vi "AH Bridge Update Int Cal.vi"(8 "error in (no error)":errorcluster, 11 "VISA resource name":refnum<visa-resource-name>) -> (0 "error out":errorcluster, 1 "Cal Done time string":string, 2 "Start time string":string, 3 "dup VISA Session":refnum<visa-resource-name>)   [LabVIEW 2025]
doc: "routine to calibrate the AH 2700 Bridge using the internal standard\nWaits for command ready status and stores calibration data, updating the calibration due date.\n\nScott Hannahs, NHMFL December 2023\n<sth@magnet.fsu.edu>\nAuthor: Scott Hannahs <sth@magnet.fsu.edu>\n\nThis software is licensed for use under the “MIT License\"\nCopyright (c) 2025 Scott Hannahs, sth@sth@magnet.sthnet.net\n\nPermission is hereby granted, free of charge, to any person obtaining a copy of this software and associated documentation files (the \"Software\"), to deal in the Software without restriction, including without limitation the rights to use, copy, modify, merge, publish, distribute, sublicense, and/or sell copies of the Software, and to permit persons to whom the Software is furnished to do so, subject to the following conditions: The above copyright notice and this permission notice shall be included in all copies or substantial portions of the Software.\n\nTHE SOFTWARE IS PROVIDED \"AS IS\", WITHOUT WARRANTY OF ANY KIND, EXPRESS OR IMPLIED, INCLUDING BUT NOT LIMITED TO THE WARRANTIES OF MERCHANTABILITY, FITNESS FOR A PARTICULAR PURPOSE AND NONINFRINGEMENT. IN NO EVENT SHALL THE AUTHORS OR COPYRIGHT HOLDERS BE LIABLE FOR ANY CLAIM, DAMAGES OR OTHER LIABILITY, WHETHER IN AN ACTION OF CONTRACT, TORT OR OTHERWISE, ARISING FROM, OUT OF OR IN CONNECTION WITH THE SOFTWARE OR THE USE OR OTHER DEALINGS IN THE SOFTWARE."
panel:
  out "status byte":u16 format="%.0b"
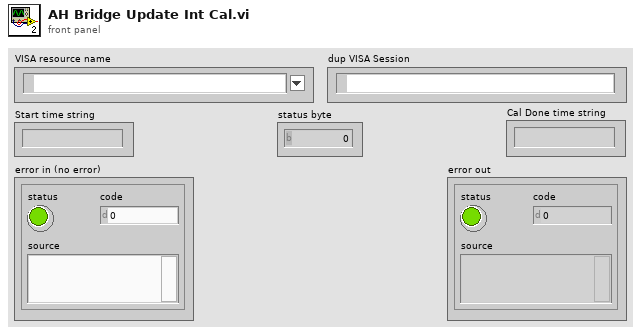
[diagram p1: front panel]
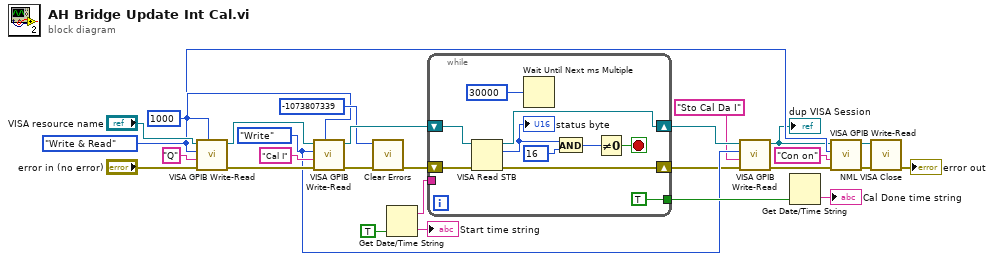
[diagram p0: block diagram]
diagram:
  w8 = u32 1000 ("Wait (ms)")
  w7 = enum16{"Write", "Read", "Write & Read"}."Write & Read" ("Action")
  w5 = enum16{"Write", "Read", "Write & Read"}."Write" ("Action")
  n1 = call "VISA GPIB Write-Read.vi"("Wait (ms)"=w8, "error in (no error)"="error in (no error)", "Command"="Q", "Action"=w7, "VISA resource name"="VISA resource name") -> ("error out"=w16:errorcluster, "dup VISA Session"=w18:refnum<visa-resource-name>)  [unwired: 3 in, 2 out]
  n2 = call "VISA GPIB Write-Read.vi"("Wait (ms)"=w8, "error in (no error)"=w16, "Command"="Cal I", "Action"=w5, "VISA resource name"=w18) -> ("error out"=w11:errorcluster, "dup VISA Session"=w22:refnum<visa-resource-name>)  [unwired: 3 in, 2 out]
  n3 = call <vilib>:"Clear Errors.vi"("error in (no error)"=w11, "specific error code to clear (0: all)"=-1073807339) -> ("error out"=w10:errorcluster)  [unwired: 4 in, 1 out]
  n4 = Get Date/Time String(want seconds? (F)=TRUE) -> (date string=w23:string, time string=→"Start time string":string)  [unwired: 2 in]
  n5 = while {
    shift-right: [w35] -> w2
    shift-left: w10 -> [w37]
    shift-right: [w34] -> w4
    shift-left: w22 -> [w36]
    tunnel: [TRUE ("want seconds? (F)")] -> w27
    tunnel: w23 -> [_]
    stop <- w30 stop-if-true
    n6 = VISA Read STB(8:w37, 11:w36) -> (0:w35:errorcluster, 2:w33:u16, 3:w34:refnum<visa-resource-name>)
    "status byte" <- w33
    n7 = Wait Until Next ms Multiple(millisecond multiple=u32 30000) -> ()  [unwired: 1 out]
    n8 = And(x=w33, y=u16 16) -> (x .and. y?=w31:u16)
    n9 = Not Equal To 0?(x=w31) -> (x != 0?=w30:bool)
  }
  n10 = call "VISA GPIB Write-Read.vi"("error in (no error)"=w2, "Command"="Sto Cal Da I", "Action"=w5, "VISA resource name"=w4) -> ("error out"=w6:errorcluster, "dup VISA Session"=w3:refnum<visa-resource-name>)  [unwired: 4 in, 2 out]
  "dup VISA Session" <- w3
  n11 = Get Date/Time String(want seconds? (F)=w27) -> (time string=→"Cal Done time string":string)  [unwired: 2 in, 1 out]
  n12 = call "VISA GPIB Write-Read.vi"("error in (no error)"=w6, "Command"="Con on", "Action"=w7, "VISA resource name"=w3) -> ("error out"=w14:errorcluster, "dup VISA Session"=w13:refnum<visa-resource-name>)  [unwired: 4 in, 2 out]
  n13 = call "NML VISA Close.vi"("Error In"=w14, "VISA resource name"=w13) -> ("Error Out"=→"error out":errorcluster)  [unwired: 9 in]
